vi "LaserUnlockNotification.vi"(11 "369wavelength":dbl) -> ()   [LabVIEW 2019]
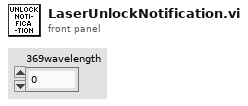
[diagram p1: front panel]
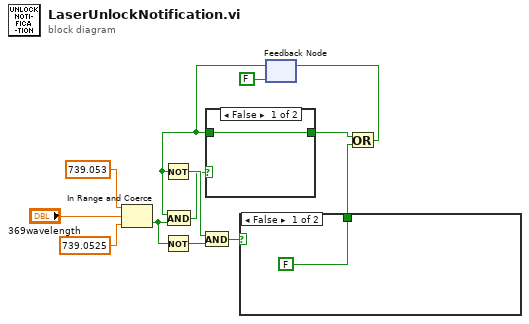
[diagram p0: block diagram]
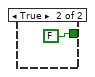
[diagram p2: hidden frame]
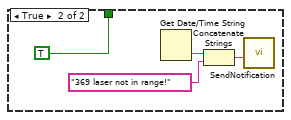
[diagram p3: hidden frame]
diagram:
  n1 = In Range and Coerce(upper limit=739.053, x="369wavelength", lower limit=739.0525) -> (In Range?=w6:bool)  [unwired: 1 out]
  n2 = Not(x=w6) -> (.not. x?=w9:bool)
  n3 = feedback #1(FALSE) -> (w4:bool)
  n4 = Not(x=w4) -> (.not. x?=w8:bool)
  n5 = And(x=w4, y=w6) -> (x .and. y?=w5:bool)
  n6 = And(x=w8, y=w9) -> (x .and. y?=w7:bool)
  n7 = case shown="False" w5 {
    tunnel: [w14 FALSE] -> w3
    tunnel: w4 -> [w14 _]
    frame False {
    }
    frame True {
    }
  }
  n8 = case shown="False" w7 {
    tunnel: [FALSE TRUE] -> w1
    frame False {
    }
    frame True {
      n9 = Get Date/Time String() -> (time string=w20:string)  [unwired: 3 in, 1 out]
      n10 = Concatenate Strings(w20, "369 laser not in range!" ("Message")) -> (w18:string)
      n11 = call "SendNotification.vi"("Message"=w18) -> ()  [unwired: 8 in, 1 out]
    }
  }
  n12 = Or(x=w3, y=w1) -> (x .or. y?=w2:bool)
  n13 = feedback-in #1(w2) -> ()
